vi "Scan Project Dependencies.vi"(5 "Img Type":T1, 6 "pattern to Include no *":string[](array[string])=["lvlib"], 7 "Working Path":path, 8 "error in":errorcluster, 9 "pattern Search":string[](array[string])=["*.lvlib"], 10 "Include vi.lib":bool, 11 "Selection":path[](array[path])) -> (0 "error out":errorcluster, 1 "Reason":T2(ring), 2 "Is Acyclic ?":bool, 3 "Dependency Plot":picture)   [LabVIEW 2020, in "SimpleDependencyInspector.lvlib"]
uses:
  SimpleDependencyInspector.lvlib
  Image Type--enum.ctl
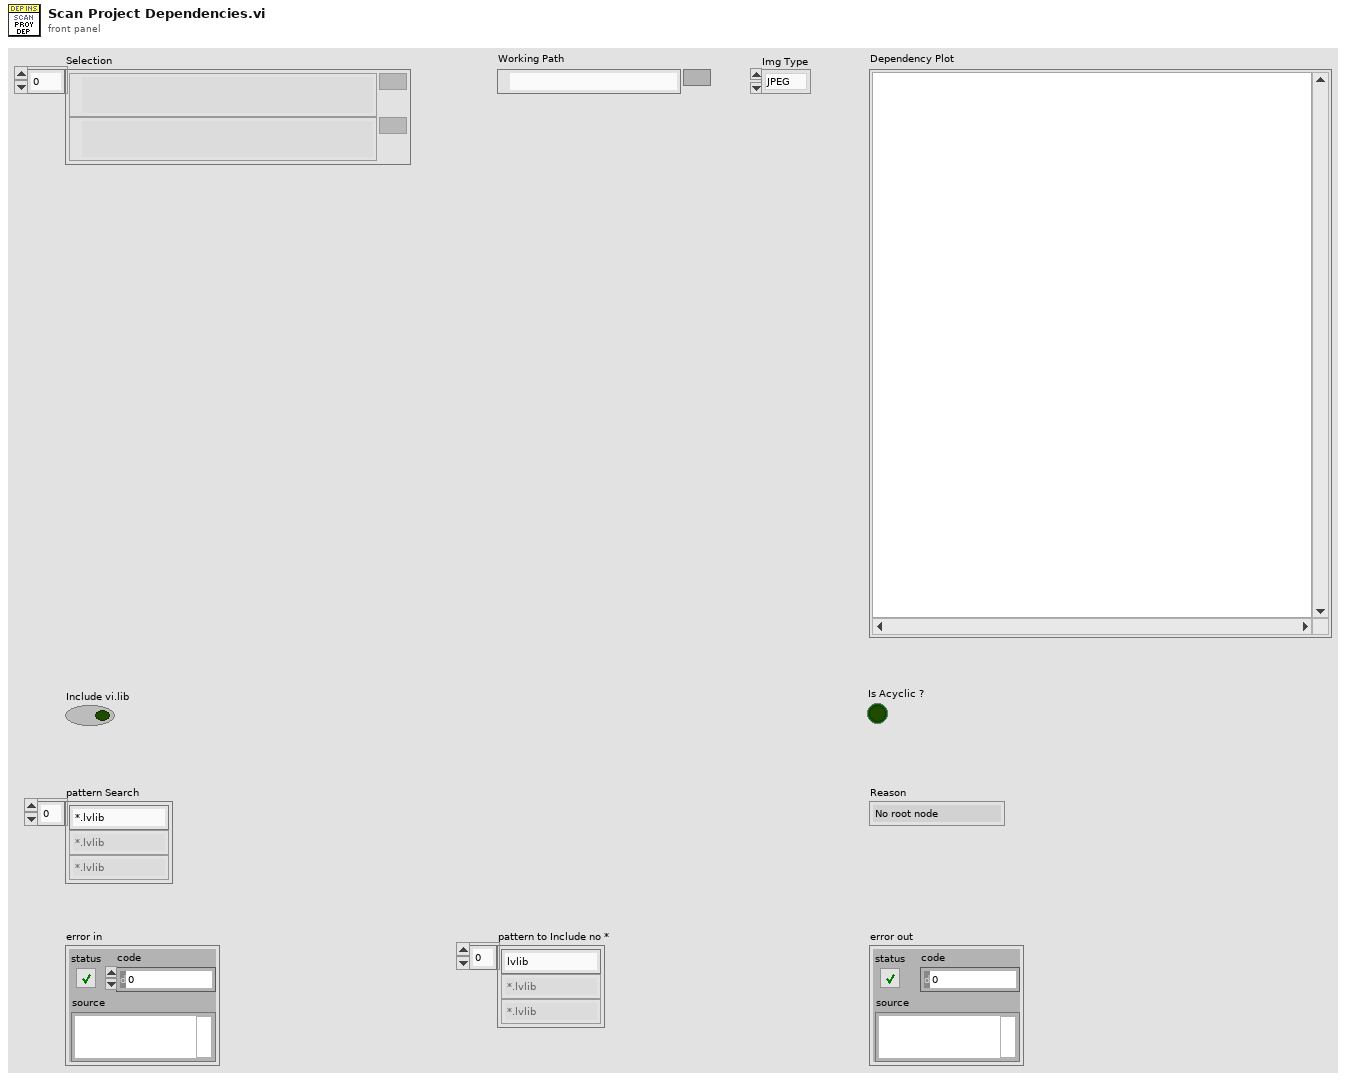
[diagram p1: front panel]
types:
  T1 = typedef "SimpleDependencyInspector.lvlib/Image Type--enum.ctl" = enum16{"JPEG", "PNG", "BMP", "SVG"}
  T2 = enum16{"No root node", "Cycle in graph", "Acyclic", "Error"}
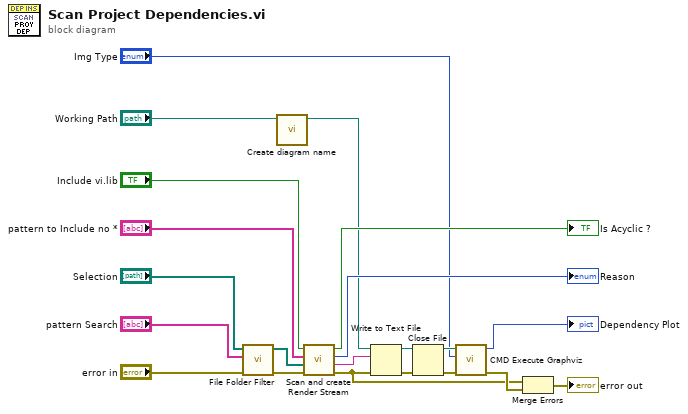
[diagram p0: block diagram]
diagram:
  n1 = call "File Folder Filter.vi"("error in"="error in", "pattern"="pattern Search", "Selection"="Selection") -> ("error out"=w20:errorcluster, "All Files in Dir"=w12:path[])  [unwired: 7 in]
  n2 = call "Create diagram name.vi"("Working Path"="Working Path") -> ("appended path"=w1:path)  [unwired: 10 in]
  n3 = call "Scan and create Render Stream.vi"("error in"=w20, "All Files in Dir"=w12, "pattern to Include no *"="pattern to Include no *", "Include vi.lib"="Include vi.lib") -> ("error out"=w15:errorcluster, "Rendered Stream"=w9:string, "Reason"=→"Reason":T2, "Is Acyclic ?"=→"Is Acyclic ?":bool)  [unwired: 4 in]
  n4 = Write to Text File(file (use dialog)=w1, text=w9, error in=w15) -> (refnum out=w8:refnum<file>, error out=w19:errorcluster)  [unwired: 1 in, 1 out]
  n5 = Close File(refnum=w8, error in=w19) -> (path=w7:path, error out=w18:errorcluster)
  n6 = call "CMD Execute Graphviz.vi"("error in"=w18, "Img Type"="Img Type", "Dot File"=w7) -> ("error out"=w17:errorcluster, "Dependency Plot"=→"Dependency Plot":picture)  [unwired: 7 in]
  n7 = Merge Errors(w15, w17) -> (→"error out":errorcluster)
